vi "ProcessName.vi"() -> (1 "ProcessName":string)   [LabVIEW 2017, in "SystemInfoProcess.lvlib"]
uses:
  <vilib>/addons/SystemInfoProcess/SystemInfoProcess.lvlib
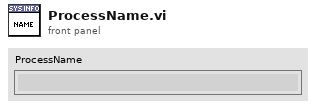
[diagram p1: front panel]
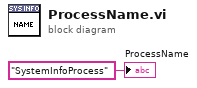
[diagram p0: block diagram]
diagram:
  "ProcessName" <- "SystemInfoProcess" ("ProcessName")
